vi "find_unused_vis.vi"() -> ()   [LabVIEW 2013]
panel:
  out "Array":string[][](array[string])
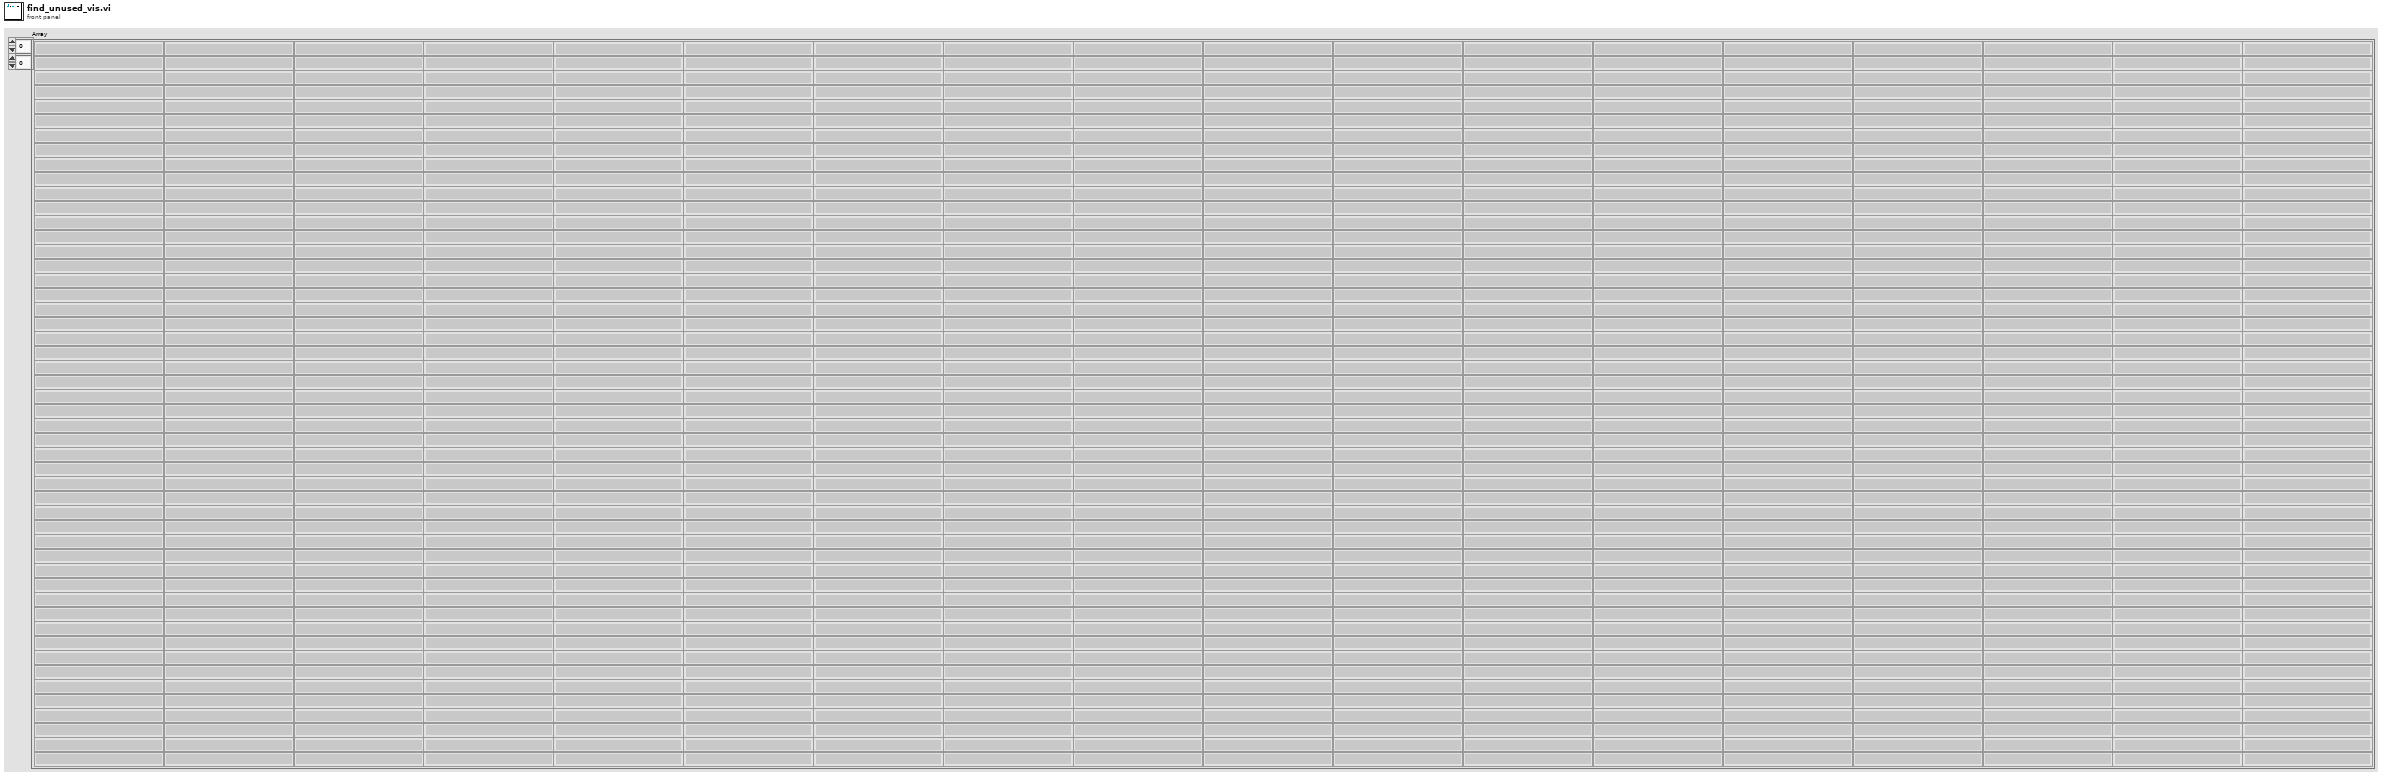
[diagram p1: front panel]
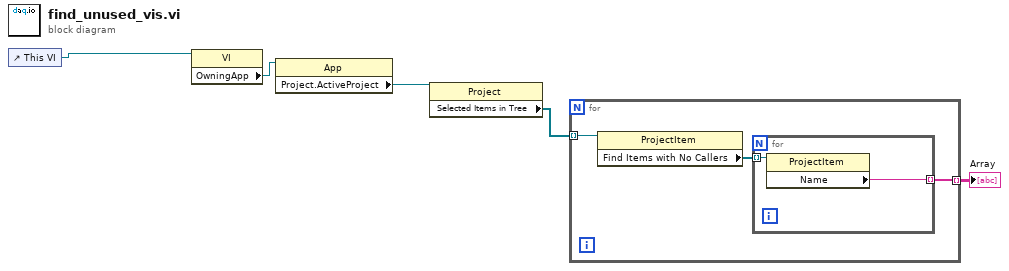
[diagram p0: block diagram]
diagram:
  n1 = control-ref of="This VI"() -> (w5:refnum<vi>)
  n2 = property class="VI"(reference=w5) -> ("OwningApp"=w4:refnum<vi>)  [unwired: 1 in, 2 out]
  n3 = property class="App"(reference=w4) -> ("Project.ActiveProject"=w3:refnum<vi>)  [unwired: 1 in, 2 out]
  n4 = property class="Project"(reference=w3) -> ("Selected Items in Tree"=w2:refnum<vi>[])  [unwired: 1 in, 2 out]
  n5 = for {
    tunnel: w2 -> [w8] mode=indexing
    tunnel: [w6] -> w1 mode=indexing
    n6 = property class="ProjectItem"(reference=w8) -> ("Find Items with No Callers"=w7:refnum<vi>[])  [unwired: 1 in, 2 out]
    n7 = for {
      tunnel: w7 -> [w10] mode=indexing
      tunnel: [w9] -> w6 mode=indexing
      n8 = property class="ProjectItem"(reference=w10) -> ("Name"=w9:string)  [unwired: 1 in, 2 out]
    }
  }
  "Array" <- w1
